vi "Get Sequences.vi"(8 "error in (no error)":errorcluster, 11 "VISA resource name":refnum<visa-resource-name>) -> (0 "error out":errorcluster, 3 "VISA resource name out":refnum<visa-resource-name>, 4 "Byte 3 Delay":u8[](array[numeric]), 5 "Byte 2 Ch.":u8[](array[numeric]), 7 "Byte 1 Ch.":u8[](array[numeric]))   [LabVIEW 2020, in "QuPMXdriver.lvlib"]
doc: "Gets all sequences from multiplexer and return bytes."
uses:
  QuPMXdriver.lvlib
  <vilib>/Utility/error.llb/Error Cluster From Error Code.vi
  <vilib>/ErrorRing/Error Ring.xnode
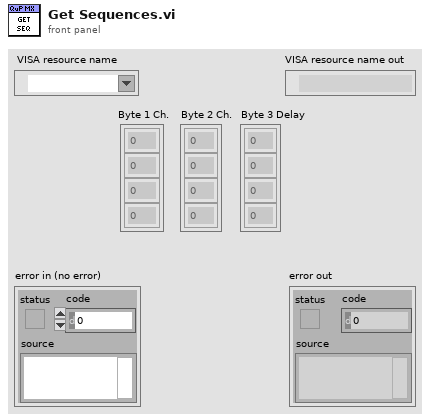
[diagram p1: front panel]
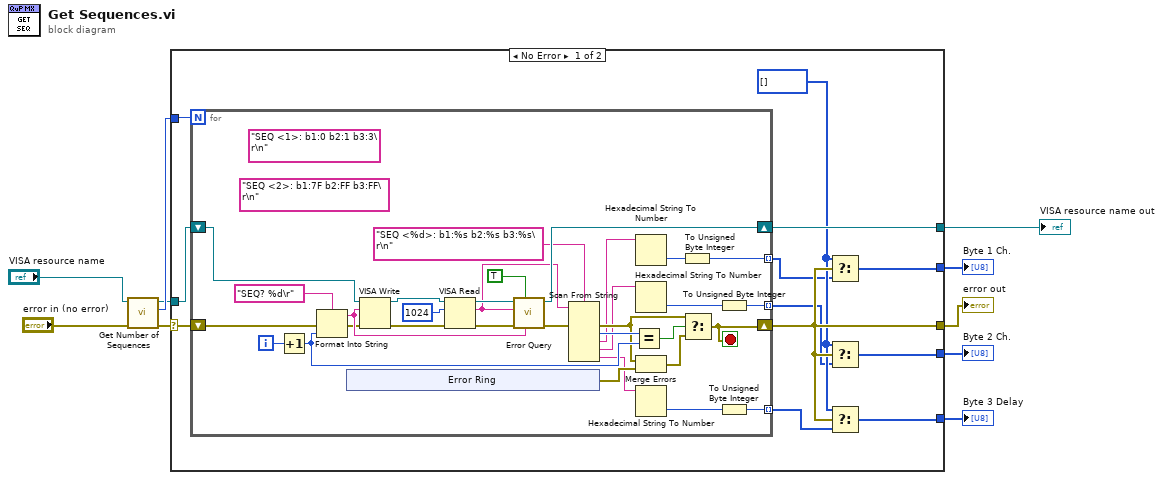
[diagram p0: block diagram]
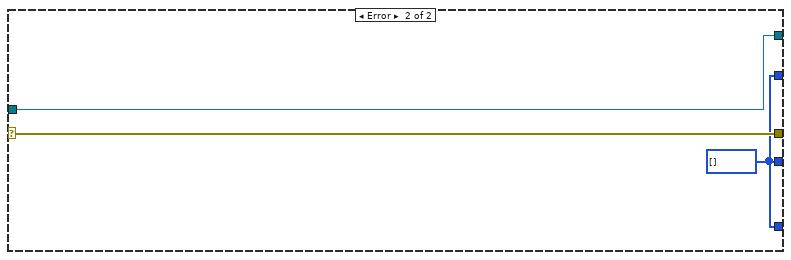
[diagram p2: hidden frame]
diagram:
  n1 = call "Get Number of Sequences.vi"("error in (no error)"="error in (no error)", "VISA resource name"="VISA resource name") -> ("error out"=w8:errorcluster, "Number of sequences"=w7:i32, "VISA resource name out"=w6:refnum<visa-resource-name>)  [unwired: 7 in]
  n2 = case shown="No Error" w8 {
    selector: w8 -> [w21 w62]
    tunnel: w7 -> [w22 _]
    tunnel: w6 -> [w20 w61]
    tunnel: [w19 w61] -> w5
    tunnel: [w18 w62] -> w4
    tunnel: [w15 w60] -> w3
    tunnel: [w16 w60] -> w2
    tunnel: [w17 w60] -> w1
    frame No Error {
      w14 = u8[] [] ("f")
      n3 = for {
        N: w22 -> [_]
        shift-right: [w34] -> w18
        shift-left: w21 -> [w45]
        shift-right: [w42] -> w19
        shift-left: w20 -> [w43]
        tunnel: [w33] -> w13 mode=indexing
        tunnel: [w32] -> w12 mode=indexing
        tunnel: [w31] -> w11 mode=indexing
        i -> [w48]
        stop <- w34 stop-if-true
        (unwired) "SEQ <2>: b1:7F b2:FF b3:FF\r\n"
        (unwired) "SEQ <1>: b1:0 b2:1 b3:3\r\n"
        n4 = Increment(x=w48) -> (x+1=w39:i32)
        n5 = Format Into String(format string="SEQ? %d\r", error in=w45, w39) -> (resulting string=w46:string, error out=w44:errorcluster)  [unwired: 1 in]
        n6 = xnode "Error Ring"() -> ("error out"=w37:errorcluster)
        n7 = VISA Write(VISA resource name=w43, write buffer=w46, error in (no error)=w44) -> (VISA resource name out=w53:refnum<visa-resource-name>, error out=w49:errorcluster)  [unwired: 1 out]
        n8 = VISA Read(VISA resource name=w53, byte count=u32 1024, error in (no error)=w49) -> (VISA resource name out=w52:refnum<visa-resource-name>, read buffer=w29:string, error out=w51:errorcluster)  [unwired: 1 out]
        n9 = call "Error Query.vi"("Last command"=w46, "Ignore empty sequence? (T)"=TRUE, "error in (no error)"=w51, "Read buffer"=w29, "VISA resource name"=w52) -> ("error out"=w41:errorcluster, "VISA resource name out"=w42:refnum<visa-resource-name>)  [unwired: 5 in]
        n10 = Scan From String(format string="SEQ <%d>: b1:%s b2:%s b3:%s\r\n", input string=w29, error in=w41) -> (error out=w36:errorcluster, output 1=w40:i32, output 2=w28:string, output 3=w26:string, output 4=w24:string)  [unwired: 5 in, 2 out]
        n11 = Equal?(x=w40, y=w39) -> (x = y?=w38:bool)
        n12 = Hexadecimal String To Number(string=w28) -> (number=w27:u32)  [unwired: 2 in, 1 out]
        n13 = Hexadecimal String To Number(string=w26) -> (number=w25:u32)  [unwired: 2 in, 1 out]
        n14 = Merge Errors(w36, w37) -> (w35:errorcluster)
        n15 = Hexadecimal String To Number(string=w24) -> (number=w23:u32)  [unwired: 2 in, 1 out]
        n16 = To Unsigned Byte Integer(number=w27) -> (unsigned 8bit integer=w33:u8)
        n17 = Select(t=w36, s=w38, f=w35) -> (s? t:f=w34:errorcluster)
        n18 = To Unsigned Byte Integer(number=w25) -> (unsigned 8bit integer=w32:u8)
        n19 = To Unsigned Byte Integer(number=w23) -> (unsigned 8bit integer=w31:u8)
      }
      n20 = Select(t=w14, s=w18, f=w13) -> (s? t:f=w15:u8[])
      n21 = Select(t=w14, s=w18, f=w12) -> (s? t:f=w16:u8[])
      n22 = Select(t=w14, s=w18, f=w11) -> (s? t:f=w17:u8[])
    }
    frame Error {
      w60 = u8[] []
    }
  }
  "error out" <- w4
  "VISA resource name out" <- w5
  "Byte 1 Ch." <- w3
  "Byte 2 Ch." <- w2
  "Byte 3 Delay" <- w1
